vi "Keithley 2450 Pulse Output List and Aquire.vi"() -> ()   [LabVIEW 2021]
doc: "Configure the measurements , output list with the amplitude array and source settings to take voltage and current readings\n\nNote:\nThis VI is only applicable to 2461 model."
uses:
  <instrlib>/Keithley 2450/Public/Data/Read (Multiple Points).vi
  <instrlib>/Keithley 2450/Keithley 2450.lvlib
panel:
  in  "Source Range (1.0)":dbl=20.0
  in  "Limit  Level (0.1)":dbl=1.0
  in  "Pulse Limit  Level (0.1)":dbl
  in  "Pulse Width":dbl=0.0002 format="%#_9g"
  in  "Pulse Off Time":dbl=0.0001 format="%#_9g"
  in  "Sample Rate (100000)":u32=2000
  in  "Measure Range (1.0)":dbl=0.1
  out "Waveform Graph":dbl[][](graph)=[[0.7197616, -0.0002586769, 1.421677, 0.01539228, -1.124387, 0.005788153, 2.743937, -0.0007559972], [0.7197616, -0.0002586769, 1.421677, 0.01539228, -1.124387, 0.005788153, 2.743937, -0.0007559972]]
  in  "Source Mode  (0: Voltage)":u16(ring) items=["Voltage", "Current"]
  in  "Output List":dbl[](array[numeric])=[1.0, 2.0, 0.0, 4.0, -3.0, 7.0, 0.0, 11.0]
  in  "VISA resource name":refnum<visa-resource-name>
  # "(c) 2021 National Instruments.  ALL RIGHTS RESERVED."
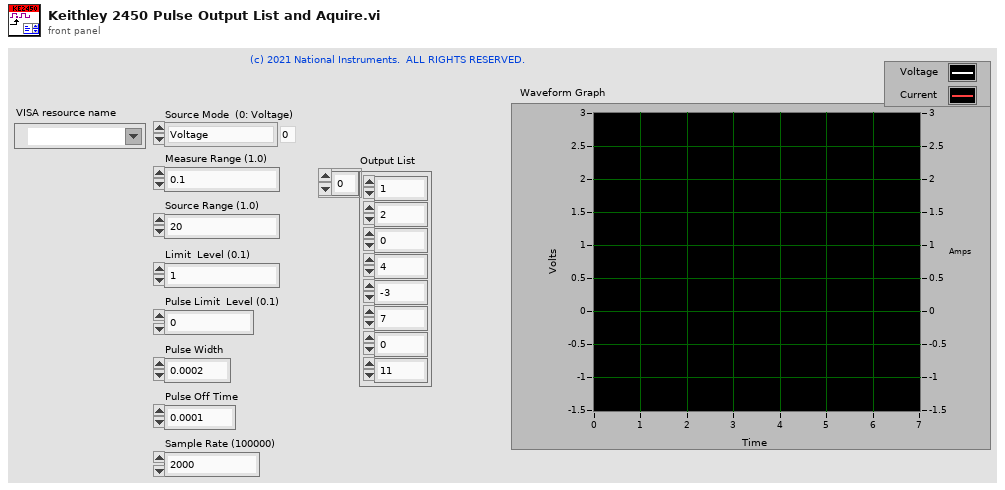
[diagram p1: front panel]
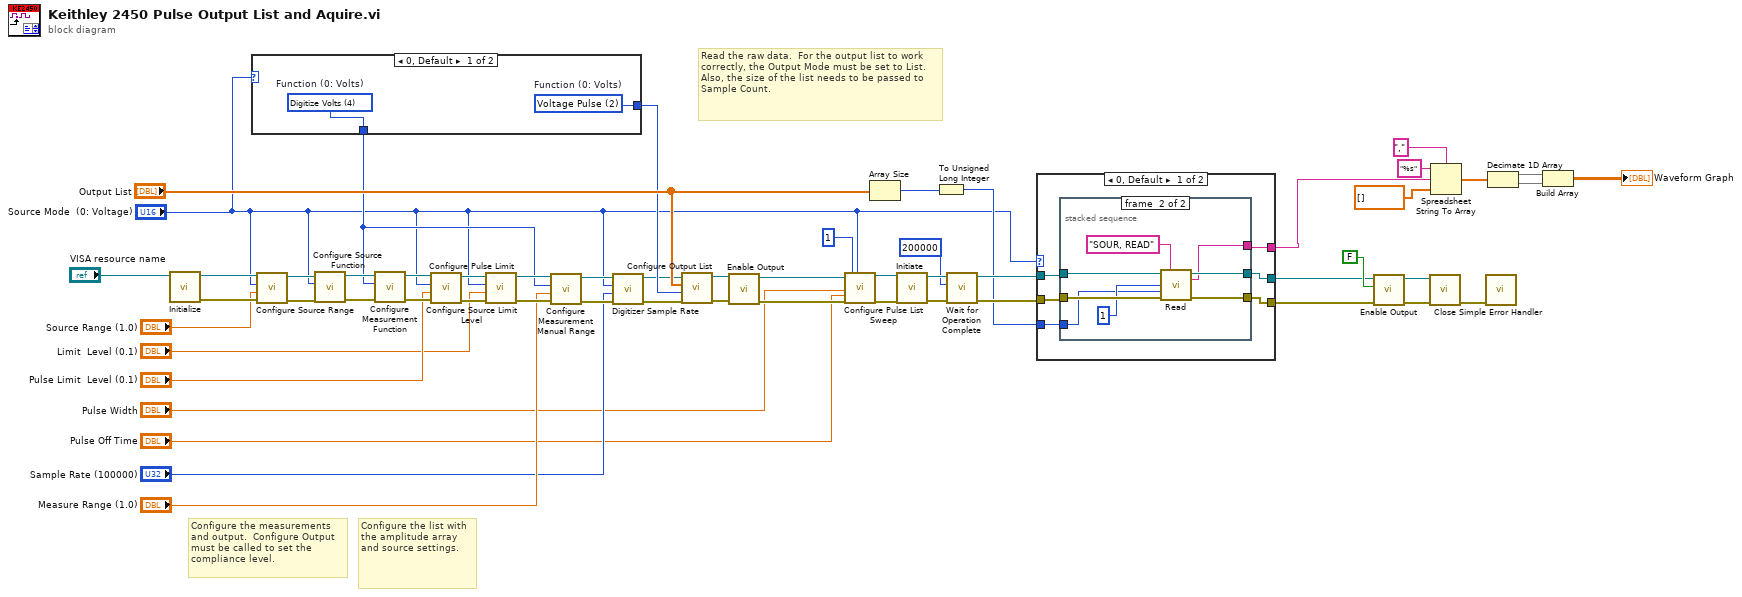
[diagram p0: block diagram]
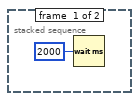
[diagram p2: hidden frame]
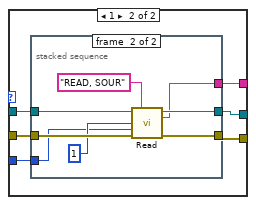
[diagram p3: hidden frame]
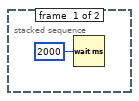
[diagram p4: hidden frame]
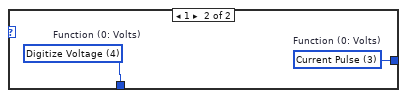
[diagram p5: hidden frame]
diagram:
  # "Read the raw data.  For the output list to work correctly, the Output Mode must be set to List.  Also, the size of the list needs to be passed to Sample Count."
  # "Configure the list with the amplitude array and source settings."
  # "Configure the measurements and output.  Configure Output must be called to set the compliance level."
  n1 = call <instrlib>:"Initialize.vi"("VISA resource name"="VISA resource name") -> ("error out"=w11:errorcluster, "VISA resource name out"=w12:refnum<visa-resource-name>)  [unwired: 9 in]
  n2 = case shown="0, Default" "Source Mode  (0: Voltage)" {
    tunnel: [w58 w60] -> w13
    tunnel: [w57 w59] -> w20
    frame 0, Default {
      w57 = u16 2 items=["Volts", "Current", "Voltage Pulse", "Current Pulse"]  # Function (0: Volts)
      w58 = u16 4 items=["Volts", "Current", "Auto Resistance", "Manual Resistance", "Digitize Volts", "Digitize Current"]  # Function (0: Volts)
    }
    frame 1 {
      w59 = u16 3 items=["Volts", "Current", "Voltage Pulse", "Current Pulse"]  # Function (0: Volts)
      w60 = u16 4 items=["Volts", "Current", "Auto Resistance", "Manual Resistance", "Digitize Voltage", "Digitize Current"]  # Function (0: Volts)
    }
  }
  n3 = call <instrlib>:"Configure Source Range.vi"("error in (no error)"=w11, "Source Range (1.0)"="Source Range (1.0)", "Function (0: Volts)"="Source Mode  (0: Voltage)", "VISA resource name"=w12) -> ("error out"=w10:errorcluster, "VISA resource name out"=w9:refnum<visa-resource-name>)  [unwired: 6 in]
  n4 = call <instrlib>:"Configure Source Function.vi"("error in (no error)"=w10, "Function (0: Volts)"="Source Mode  (0: Voltage)", "VISA resource name"=w9) -> ("error out"=w36:errorcluster, "VISA resource name out"=w37:refnum<visa-resource-name>)  [unwired: 7 in]
  n5 = call <instrlib>:"Configure Measurement Function.vi"("error in (no error)"=w36, "Function (0: Volts)"=w13, "VISA resource name"=w37) -> ("error out"=w28:errorcluster, "VISA resource name out"=w29:refnum<visa-resource-name>)  [unwired: 7 in]
  n6 = call <instrlib>:"Configure Pulse Limit.vi"("error in (no error)"=w28, "Limit"="Pulse Limit  Level (0.1)", "Function (0:Voltage)"="Source Mode  (0: Voltage)", "VISA resource name"=w29) -> ("error out"=w26:errorcluster, "VISA resource name out"=w27:refnum<visa-resource-name>)  [unwired: 6 in]
  n7 = call <instrlib>:"Configure Source Limit Level.vi"("error in (no error)"=w26, "Source Limit (1.0)"="Limit  Level (0.1)", "Function (0: Volts)"="Source Mode  (0: Voltage)", "VISA resource name"=w27) -> ("error out"=w16:errorcluster, "VISA resource name out"=w17:refnum<visa-resource-name>)  [unwired: 6 in]
  n8 = call <instrlib>:"Configure Measurement Manual Range.vi"("error in (no error)"=w16, "Manual Range (1.0)"="Measure Range (1.0)", "Function (0: Volts)"=w13, "VISA resource name"=w17) -> ("error out"=w15:errorcluster, "VISA resource name out"=w14:refnum<visa-resource-name>)  [unwired: 6 in]
  n9 = call <instrlib>:"Digitizer Sample Rate.vi"("error in (no error)"=w15, "Sample Rate (100000)"="Sample Rate (100000)", "Digitize Function (Voltage)"="Source Mode  (0: Voltage)", "VISA resource name"=w14) -> ("error out"=w19:errorcluster, "VISA resource name out"=w18:refnum<visa-resource-name>)  [unwired: 6 in]
  n10 = call <instrlib>:"Configure Output List.vi"("error in (no error)"=w19, "Source Mode  (0: Voltage)"=w20, "Output List"="Output List", "VISA resource name"=w18) -> ("error out"=w53:errorcluster, "VISA resource name out"=w54:refnum<visa-resource-name>)  [unwired: 6 in]
  n11 = call <instrlib>:"Enable Output.vi"("error in (no error)"=w53, "VISA resource name"=w54) -> ("error out"=w23:errorcluster, "VISA resource name out"=w22:refnum<visa-resource-name>)  [unwired: 8 in]
  n12 = call <instrlib>:"Configure Pulse List Sweep.vi"("VISA resource name"=w22, "Pulse Width"="Pulse Width", "Pulse Off Time"="Pulse Off Time", "error in (no error)"=w23, "Start Index (1)"=u32 1 ("Start Index"), "Source Mode  (0: Voltage)"="Source Mode  (0: Voltage)") -> ("VISA resource name out"=w25:refnum<visa-resource-name>, "error out"=w24:errorcluster)  [unwired: 12 in]
  n13 = Array Size(array="Output List") -> (size(s)=w49:i32)
  n14 = call <instrlib>:"Initiate.vi"("error in (no error)"=w24, "VISA resource name"=w25) -> ("error out"=w39:errorcluster, "VISA resource name out"=w40:refnum<visa-resource-name>)  [unwired: 8 in]
  n15 = To Unsigned Long Integer(number=w49) -> (unsigned 32bit integer=w30:u32)
  n16 = call <instrlib>:"Wait for Operation Complete.vi"("error in (no error)"=w39, "Timeout (10000 ms)"=200000, "VISA resource name"=w40) -> ("error out"=w34:errorcluster, "VISA resource name out"=w35:refnum<visa-resource-name>)  [unwired: 7 in]
  n17 = case shown="0, Default" "Source Mode  (0: Voltage)" {
    tunnel: w35 -> [w66 w81]
    tunnel: w34 -> [w65 w80]
    tunnel: [w64 w78] -> w33
    tunnel: [w63 w77] -> w32
    tunnel: w30 -> [w62 w79]
    tunnel: [w61 w76] -> w31
    frame 0, Default {
      n18 = stacked-sequence {
        tunnel: [_ w75] -> w64
        tunnel: [_ w74] -> w63
        tunnel: w66 -> [_ w72]
        tunnel: w65 -> [_ w71]
        tunnel: [_ w70] -> w61
        tunnel: w62 -> [_ w68]
        frame #0 {
          n19 = Wait (ms)(milliseconds to wait=u32 2000) -> ()  [unwired: 1 out]
        }
        frame #1 {
          n20 = call-poly <instrlib>:"Read.vi"("VISA resource name"=w72, "Buffer Elements"="SOUR, READ", "Start Index (1)"=1, "End Index (1)"=w68, "error in (no error)"=w71) -> ("VISA resource name out"=w75:refnum<visa-resource-name>, "Data out"=w70:string, "error out"=w74:errorcluster)  [unwired: 8 in]
        }
      }
    }
    frame 1 {
      n21 = stacked-sequence {
        tunnel: [_ w90] -> w78
        tunnel: [_ w89] -> w77
        tunnel: w81 -> [_ w87]
        tunnel: w80 -> [_ w86]
        tunnel: [_ w85] -> w76
        tunnel: w79 -> [_ w83]
        frame #0 {
          n22 = Wait (ms)(milliseconds to wait=u32 2000) -> ()  [unwired: 1 out]
        }
        frame #1 {
          n23 = call-poly <instrlib>:"Read.vi"("VISA resource name"=w87, "Buffer Elements"="READ, SOUR", "Start Index (1)"=1, "End Index (1)"=w83, "error in (no error)"=w86) -> ("VISA resource name out"=w90:refnum<visa-resource-name>, "Data out"=w85:string, "error out"=w89:errorcluster)  [unwired: 8 in]
        }
      }
    }
  }
  n24 = call <instrlib>:"Enable Output.vi"("error in (no error)"=w32, "Enable Output (T: Enable)"=FALSE, "VISA resource name"=w33) -> ("error out"=w52:errorcluster, "VISA resource name out"=w51:refnum<visa-resource-name>)  [unwired: 7 in]
  n25 = call <instrlib>:"Close.vi"("error in (no error)"=w52, "VISA resource name"=w51) -> ("error out"=w55:errorcluster)  [unwired: 9 in]
  n26 = Spreadsheet String To Array(delimiter (Tab)=",", format string="%s", spreadsheet string=w31, array type (2D Dbl)=dbl[] []) -> (array=w45:dbl[])
  n27 = call <vilib>:"Simple Error Handler.vi"("error in (no error)"=w55) -> ()  [unwired: 4 in, 5 out]
  n28 = Decimate 1D Array(w45) -> (w44:dbl[], w43:dbl[])
  n29 = Build Array(w44, w43) -> (→"Waveform Graph":dbl[][])
